vi "QTrkBuildLUTPlaneFromFrame.vi"(0 "QTrk Instance":T1, 5 "Image":T2, 7 "flags":u32, 9 "plane":i32, 12 "ROI Positions (corner-based)":cluster{"X":i32, "Y":i32}[](array[cluster])) -> (4 "QTrk Instance":T1)   [LabVIEW 2011]
uses:
  QTrkInstance.ctl
  <vilib>/vision/Image Controls.llb/IMAQ Image.ctl
panel:
  # "Takes a full captured IMAQ Image, cuts out ROIs and uses \" build lut plane \" to send to QTrk"
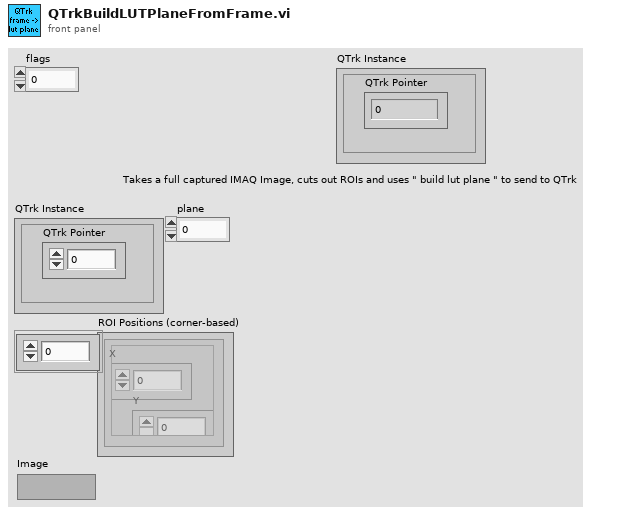
[diagram p1: front panel]
types:
  T1 = typedef "QTrkInstance.ctl" = cluster{"QTrk Pointer":u64}
  T2 = typedef "IMAQ Image.ctl" = refnum<image>
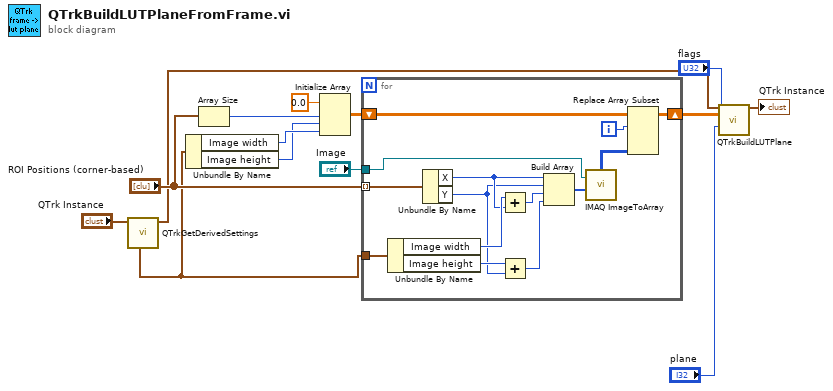
[diagram p0: block diagram]
diagram:
  n1 = call "QTrkGetDerivedSettings.vi"("QTrk Instance"="QTrk Instance") -> ("QTrk Instance (out)"=w3:T1, "ROI size"=w2:cluster{"Image width":i32, "Image height":i32})  [unwired: 5 in, 4 out]
  n2 = Unbundle By Name(w2) -> ("Image width"=w11:i32, "Image height"=w10:i32)
  n3 = Array Size(array="ROI Positions (corner-based)") -> (size(s)=w8:i32)
  n4 = Initialize Array(sgl 0.0 ("element"), w8, w10, w11) -> (w7:sgl[][][])
  n5 = for {
    tunnel: "ROI Positions (corner-based)" -> [w27] mode=indexing
    tunnel: "Image" -> [w28]
    tunnel: w2 -> [w19]
    shift-right: [w17] -> w6
    shift-left: w7 -> [w18]
    i -> [w16]
    n6 = Unbundle By Name(w19) -> ("Image width"=w26:i32, "Image height"=w24:i32)
    n7 = Unbundle By Name(w27) -> ("X"=w25:i32, "Y"=w22:i32)
    n8 = Add(x=w26, y=w25) -> (x+y=w23:i32)
    n9 = Add(x=w24, y=w22) -> (x+y=w21:i32)
    n10 = Build Array(w25, w22, w23, w21) -> (w20:i32[])
    n11 = call "IMAQ ImageToArray"("Optional Rectangle"=w20, "Image"=w28) -> ("Image Pixels (U8)"=w15:u8[][])  [unwired: 2 in, 4 out]
    n12 = Replace Array Subset(array=w18, new element=w15, index (dim 0)=w16) -> (w17:sgl[][][])  [unwired: 2 in]
  }
  n13 = call "QTrkBuildLUTPlane.vi"("QTrk Instance"=w3, "Bead images"=w6, "flags"="flags", "plane"="plane") -> ("QTrk Instance"=→"QTrk Instance":T1)  [unwired: 10 in, 1 out]
